vi "test-timer-all.vi"(8 "error in (no error)":errorcluster) -> (0 "error out":errorcluster, 3 "ALL TESTS PASSED":bool)   [LabVIEW 2019]
uses:
  <vilib>/Utility/semaphor.llb/Obtain Semaphore Reference.vi
  <vilib>/Rock Robotics/WPI/ThirdParty/JAS_Junk/TrajLib/Trajectory_Library.lvlib
panel:
  out "error out 2":errorcluster
  out "T5 - 2   0.500":dbl
  out "T5 Passed":bool
  out "T5 - 1":dbl
  out "T5 - 0":dbl
  out "T4 - 6 FALSE":bool
  out "T4 - 4 TRUE":bool
  out "T4 - 5 TRUE":bool
  out "T4 - 2 TRUE":bool
  out "T4 - 3 FALSE":bool
  out "T4 - 1 FALSE":bool
  out "T4 - 0 FALSE":bool
  out "T4 Passed":bool
  out "T3 Passed":bool
  out "T3-3 -- 0.0":dbl
  out "T3-2 -- 0.5":dbl
  out "T3-1 -- 0.0":dbl
  out "T3-0 -- 0.5":dbl
  out "Expired 2":bool
  out "Expired":bool
  out "T2 After Start":dbl
  out "Passed 2":bool
  out "T1 After Stop":dbl
  out "T1 After Start":dbl
  out "Passed 0A":bool
  out "Passed 0":bool
  out "T0 - Diff = 5.0":dbl
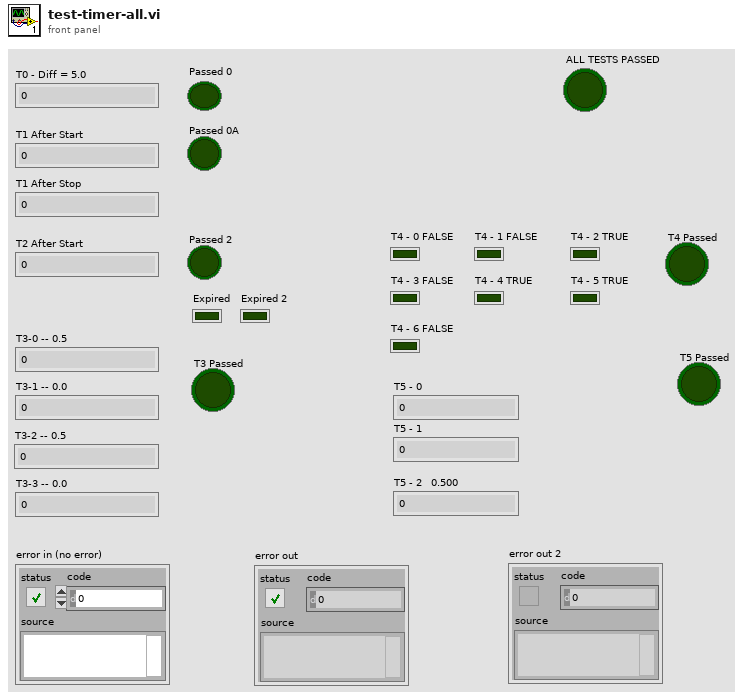
[diagram p1: front panel]
types:
  T1 = typedef "Trajectory_Library.lvlib/TIMER.ctl" = cluster{"StartTime":dbl, "Accumulated TIme":dbl, "Running":bool, "semaphore":T2}
  T2 = typedef "Semaphore RefNum" = refnum<k1>
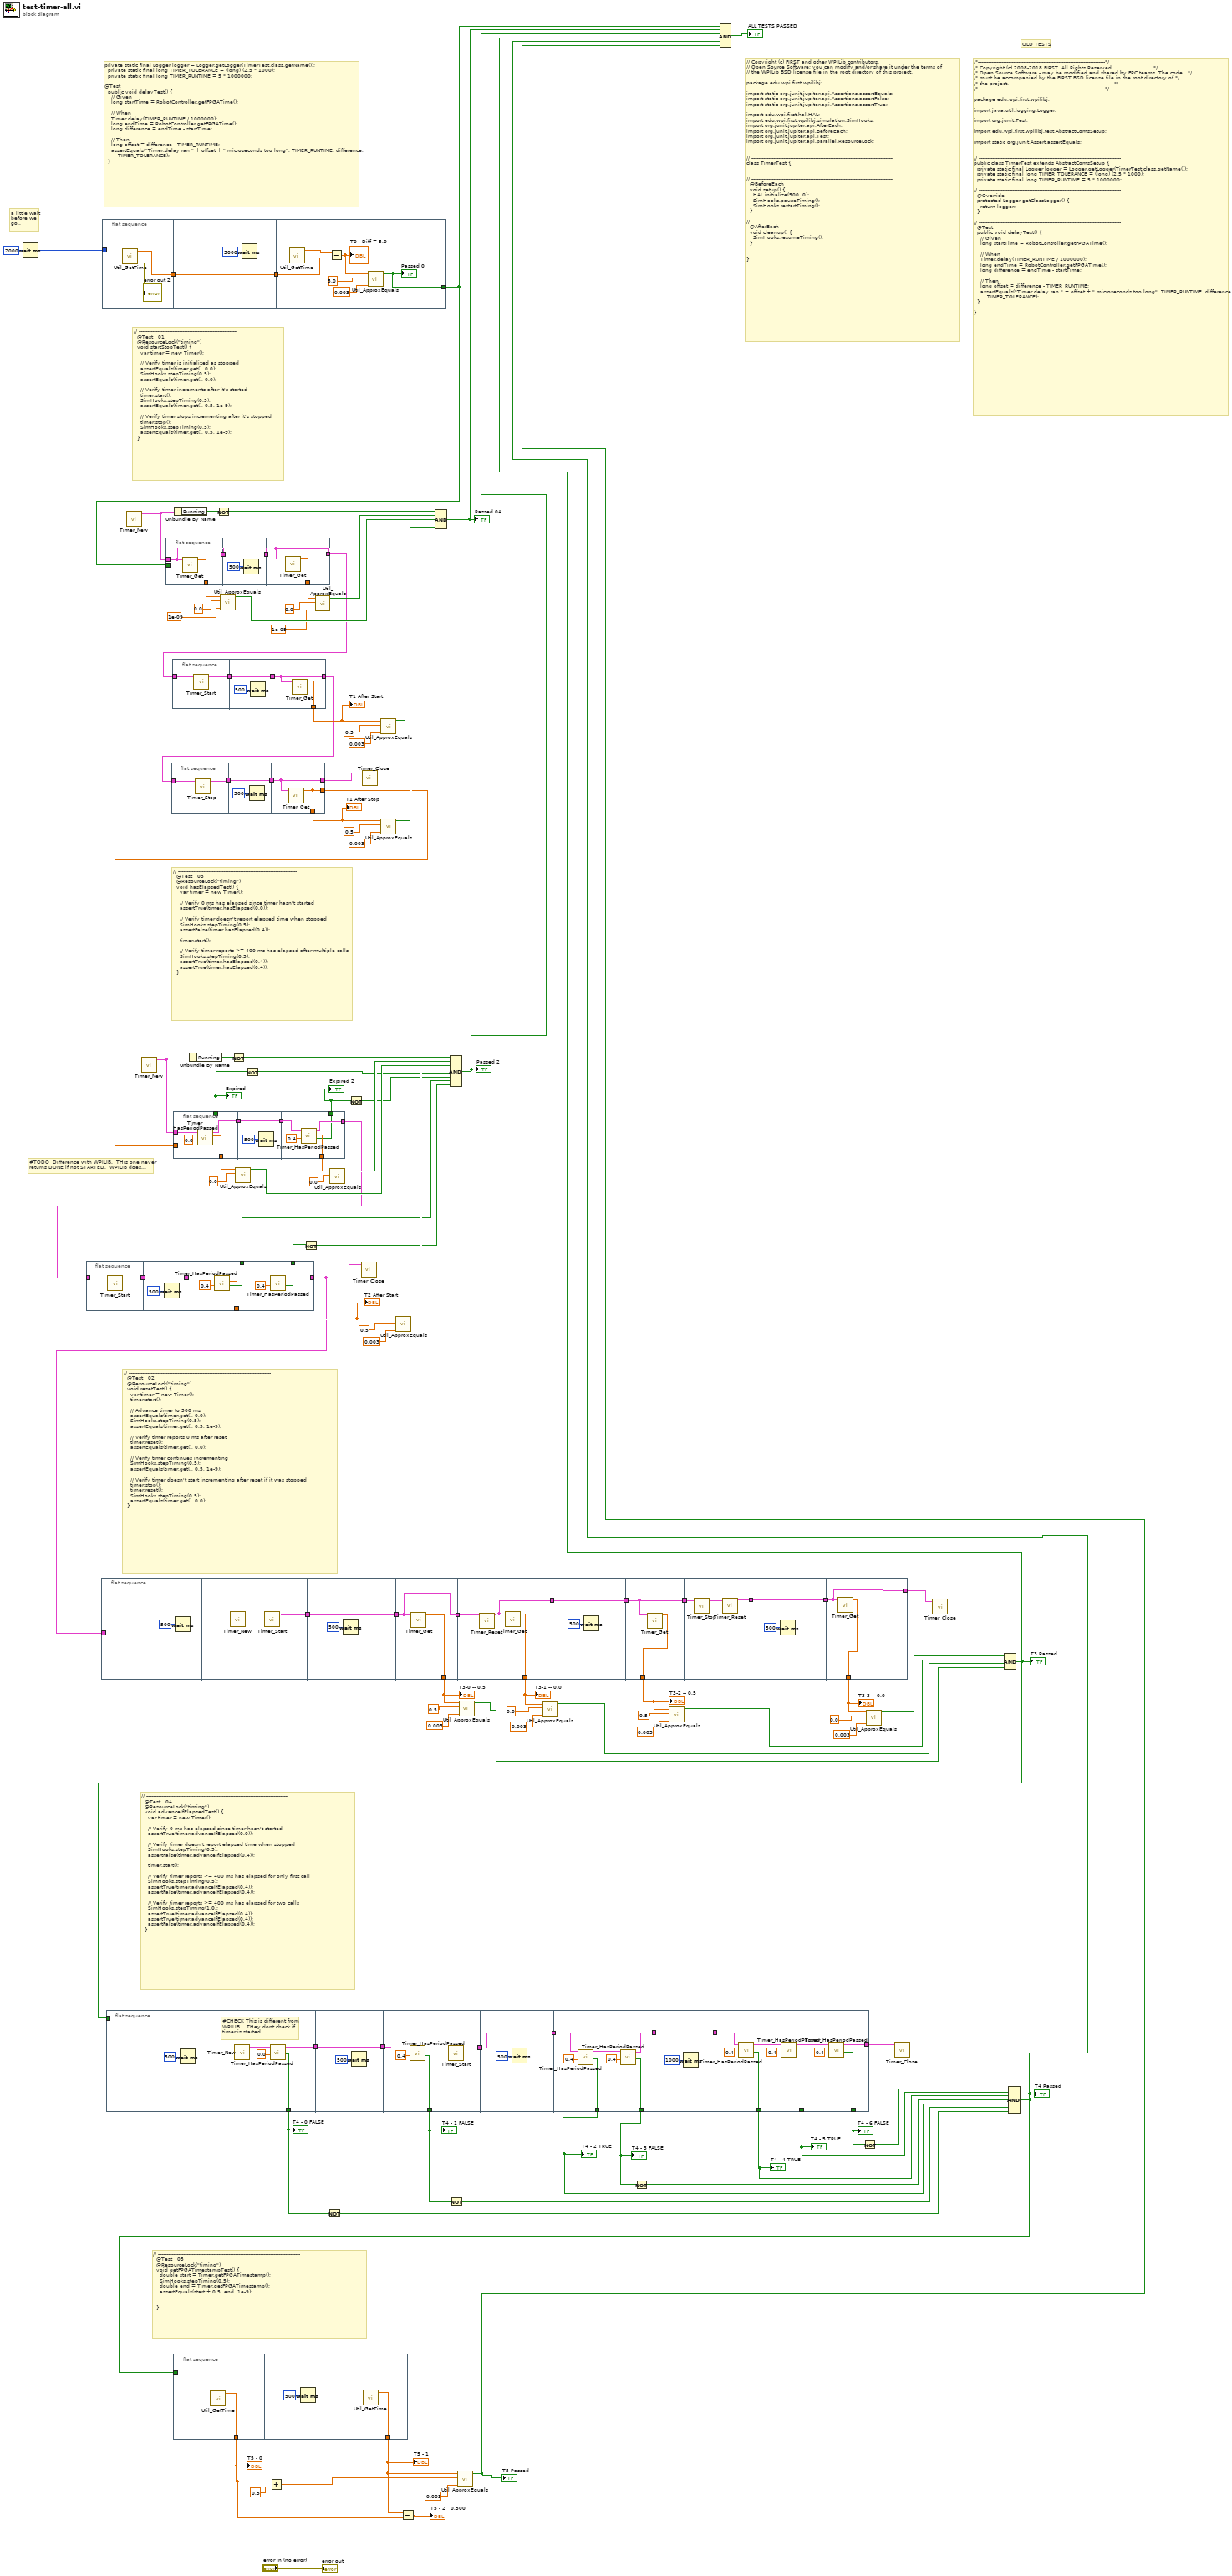
[diagram p0: block diagram]
diagram:
  # "// -------------------------------------------------------------------------------------\n  @Test   05\n  @ResourceLock(\"timing\")\n  void getFPGATimestampTest() {\n    double start = Timer.getFPGATimestamp();\n    SimHooks.stepTiming(0.5);\n    double end = Timer.getFPGATimestamp();\n    assertEquals(start + 0.5, end, 1e-9);\n\n\n  }"
  # "OLD TESTS"
  # "// -------------------------------------------------------------------------------------\n  @Test   04\n  @ResourceLock(\"timing\")\n  void advanceIfElapsedTest() {\n    var timer = new Timer();\n\n    // Verify 0 ms has elapsed since timer hasn't started\n    assertTrue(timer.advanceIfElapsed(0.0));\n\n    // Verify timer doesn't report elapsed time when stopped\n    SimHooks.stepTiming(0.5);\n    assertFalse(timer.advanceIfElapsed(0.4));\n\n    timer.start();\n\n    // Verify timer reports >= 400 ms has elapsed for only first call\n    SimHooks.stepTiming(0.5);\n    assertTrue(timer.advanceIfElapsed(0.4));\n    assertFalse(timer.advanceIfElapsed(0.4));\n\n    // Verify timer reports >= 400 ms has elapsed for two calls\n    SimHooks.stepTiming(1.0);\n    assertTrue(timer.advanceIfElapsed(0.4));\n    assertTrue(timer.advanceIfElapsed(0.4));\n    assertFalse(timer.advanceIfElapsed(0.4));\n  }"
  # "a little wait\nbefore we\ngo.."
  # "// -------------------------------------------------------------------------------------\n  @Test   02\n  @ResourceLock(\"timing\")\n  void resetTest() {\n    var timer = new Timer();\n    timer.start();\n\n    // Advance timer to 500 ms\n    assertEquals(timer.get(), 0.0);\n    SimHooks.stepTiming(0.5);\n    assertEquals(timer.get(), 0.5, 1e-9);\n\n    // Verify timer reports 0 ms after reset\n    timer.reset();\n    assertEquals(timer.get(), 0.0);\n\n    // Verify timer continues incrementing\n    SimHooks.stepTiming(0.5);\n    assertEquals(timer.get(), 0.5, 1e-9);\n\n    // Verify timer doesn't start incrementing after reset if it was stopped\n    timer.stop();\n    timer.reset();\n    SimHooks.stepTiming(0.5);\n    assertEquals(timer.get(), 0.0);\n  }"
  # "#TODO  Difference with WPILIB.  THis one never\nreturns DONE if not STARTED.  WPILIB does..."
  # "// -----------------------------------------------------------------------\n  @Test   03\n  @ResourceLock(\"timing\")\n  void hasElapsedTest() {\n    var timer = new Timer();\n\n    // Verify 0 ms has elapsed since timer hasn't started\n    assertTrue(timer.hasElapsed(0.0));\n\n    // Verify timer doesn't report elapsed time when stopped\n    SimHooks.stepTiming(0.5);\n    assertFalse(timer.hasElapsed(0.4));\n\n    timer.start();\n\n    // Verify timer reports >= 400 ms has elapsed after multiple calls\n    SimHooks.stepTiming(0.5);\n    assertTrue(timer.hasElapsed(0.4));\n    assertTrue(timer.hasElapsed(0.4));\n  }"
  # "// -----------------------------------------------------------\n  @Test   01\n  @ResourceLock(\"timing\")\n  void startStopTest() {\n    var timer = new Timer();\n\n    // Verify timer is initialized as stopped\n    assertEquals(timer.get(), 0.0);\n    SimHooks.stepTiming(0.5);\n    assertEquals(timer.get(), 0.0);\n\n    // Verify timer increments after it's started\n    timer.start();\n    SimHooks.stepTiming(0.5);\n    assertEquals(timer.get(), 0.5, 1e-9);\n\n    // Verify timer stops incrementing after it's stopped\n    timer.stop();\n    SimHooks.stepTiming(0.5);\n    assertEquals(timer.get(), 0.5, 1e-9);\n  }"
  # "/*----------------------------------------------------------------------------*/\n/* Copyright (c) 2008-2018 FIRST. All Rights Reserved.                        */\n/* Open Source Software - may be modified and shared by FRC teams. The code   */\n/* must be accompanied by the FIRST BSD license file in the root directory of */\n/* the project.                                                               */\n/*----------------------------------------------------------------------------*/\n\npackage edu.wpi.first.wpilibj;\n\nimport java.util.logging.Logger;\n\nimport org.junit.Test;\n\nimport edu.wpi.first.wpilibj.test.AbstractComsSetup;\n\nimport static org.junit.Assert.assertEquals;\n\n\n// -------------------------------------------------------------------------------------\npublic class TimerTest extends AbstractComsSetup {\n  private static final Logger logger = Logger.getLogger(TimerTest.class.getName());\n  private static final long TIMER_TOLERANCE = (long) (2.5 * 1000);\n  private static final long TIMER_RUNTIME = 5 * 1000000;\n\n// -------------------------------------------------------------------------------------\n  @Override\n  protected Logger getClassLogger() {\n    return logger;\n  }\n\n// -------------------------------------------------------------------------------------\n  @Test\n  public void delayTest() {\n    // Given\n    long startTime = RobotController.getFPGATime();\n\n    // When\n    Timer.delay(TIMER_RUNTIME / 1000000);\n    long endTime = RobotController.getFPGATime();\n    long difference = endTime - startTime;\n\n    // Then\n    long offset = difference - TIMER_RUNTIME;\n    assertEquals(\"Timer.delay ran \" + offset + \" microseconds too long\", TIMER_RUNTIME, difference,\n        TIMER_TOLERANCE);\n  }\n\n}"
  # "// Copyright (c) FIRST and other WPILib contributors.\n// Open Source Software; you can modify and/or share it under the terms of\n// the WPILib BSD license file in the root directory of this project.\n\npackage edu.wpi.first.wpilibj;\n\nimport static org.junit.jupiter.api.Assertions.assertEquals;\nimport static org.junit.jupiter.api.Assertions.assertFalse;\nimport static org.junit.jupiter.api.Assertions.assertTrue;\n\nimport edu.wpi.first.hal.HAL;\nimport edu.wpi.first.wpilibj.simulation.SimHooks;\nimport org.junit.jupiter.api.AfterEach;\nimport org.junit.jupiter.api.BeforeEach;\nimport org.junit.jupiter.api.Test;\nimport org.junit.jupiter.api.parallel.ResourceLock;\n\n\n// -------------------------------------------------------------------------------------\nclass TimerTest {\n\n\n// -------------------------------------------------------------------------------------\n  @BeforeEach\n  void setup() {\n    HAL.initialize(500, 0);\n    SimHooks.pauseTiming();\n    SimHooks.restartTiming();\n  }\n\n// -------------------------------------------------------------------------------------\n  @AfterEach\n  void cleanup() {\n    SimHooks.resumeTiming();\n  }\n\n\n}"
  # "private static final Logger logger = Logger.getLogger(TimerTest.class.getName());\n  private static final long TIMER_TOLERANCE = (long) (2.5 * 1000);\n  private static final long TIMER_RUNTIME = 5 * 1000000;\n\n@Test\n  public void delayTest() {\n    // Given\n    long startTime = RobotController.getFPGATime();\n\n    // When\n    Timer.delay(TIMER_RUNTIME / 1000000);\n    long endTime = RobotController.getFPGATime();\n    long difference = endTime - startTime;\n\n    // Then\n    long offset = difference - TIMER_RUNTIME;\n    assertEquals(\"Timer.delay ran \" + offset + \" microseconds too long\", TIMER_RUNTIME, difference,\n        TIMER_TOLERANCE);\n  }"
  n1 = Wait (ms)(milliseconds to wait=u32 2000) -> (millisecond timer value=w58:u32)
  n2 = flat-sequence {
    tunnel: w76 -> [w118]
    tunnel: [w117] -> w86
    tunnel: [w119] -> w85
    tunnel: w86 -> [w119]
    tunnel: [w121] -> w74
    tunnel: w85 -> [w128]
    tunnel: [w126] -> w57
    tunnel: [w123] -> w65
    tunnel: [w122] -> w64
    frame #0 {
      n3 = call <vilib>:"Timer_Start.vi"("in Timer"=w118) -> ("out Timer"=w117:T1)  [unwired: 10 in]
    }
    frame #1 {
      n4 = Wait (ms)(milliseconds to wait=u32 500) -> ()  [unwired: 1 out]
    }
    frame #2 {
      n5 = call <vilib>:"Timer_HasPeriodPassed.vi"("Period"=0.4, "in Timer"=w128) -> ("Expired"=w123:bool, "CurrentTImer"=w121:dbl, "out Timer"=w127:T1)  [unwired: 7 in]
      n6 = call <vilib>:"Timer_HasPeriodPassed.vi"("Period"=0.4, "in Timer"=w127) -> ("Expired"=w122:bool, "out Timer"=w126:T1)  [unwired: 7 in, 1 out]
    }
  }
  n7 = flat-sequence {
    tunnel: w57 -> [_]
    tunnel: [w130] -> w56
    tunnel: w56 -> [w132]
    tunnel: [w132] -> w55
    tunnel: w55 -> [w135]
    tunnel: [w135] -> w54
    tunnel: [w134] -> w51
    tunnel: w54 -> [w138]
    tunnel: [w137] -> w49
    tunnel: [w136] -> w46
    tunnel: [w139] -> w47
    tunnel: w46 -> [w139]
    tunnel: w47 -> [w141]
    tunnel: [w142] -> w43
    tunnel: [w141] -> w42
    tunnel: w42 -> [w144]
    tunnel: [w143] -> w40
    tunnel: [w146] -> w41
    tunnel: w40 -> [w146]
    tunnel: w41 -> [w148]
    tunnel: [w149] -> w37
    tunnel: [w148] -> w35
    frame #0 {
      n8 = Wait (ms)(milliseconds to wait=u32 500) -> ()  [unwired: 1 out]
    }
    frame #1 {
      n9 = call <vilib>:"Timer_New.vi"() -> ("TIMER"=w131:T1)  [unwired: 11 in]
      n10 = call <vilib>:"Timer_Start.vi"("in Timer"=w131) -> ("out Timer"=w130:T1)  [unwired: 10 in]
    }
    frame #2 {
      n11 = Wait (ms)(milliseconds to wait=u32 500) -> ()  [unwired: 1 out]
    }
    frame #3 {
      n12 = call <vilib>:"Timer_Get.vi"("TIMER"=w135) -> ("CurrentTImer"=w134:dbl)  [unwired: 10 in]
    }
    frame #4 {
      n13 = call <vilib>:"Timer_Reset.vi"("in TIMER"=w138) -> ("out TIMER"=w136:T1)  [unwired: 10 in]
      n14 = call <vilib>:"Timer_Get.vi"("TIMER"=w136) -> ("CurrentTImer"=w137:dbl)  [unwired: 10 in]
    }
    frame #5 {
      n15 = Wait (ms)(milliseconds to wait=u32 500) -> ()  [unwired: 1 out]
    }
    frame #6 {
      n16 = call <vilib>:"Timer_Get.vi"("TIMER"=w141) -> ("CurrentTImer"=w142:dbl)  [unwired: 10 in]
    }
    frame #7 {
      n17 = call <vilib>:"Timer_Stop.vi"("in Timer"=w144) -> ("out Timer"=w145:T1)  [unwired: 10 in]
      n18 = call <vilib>:"Timer_Reset.vi"("in TIMER"=w145) -> ("out TIMER"=w143:T1)  [unwired: 10 in]
    }
    frame #8 {
      n19 = Wait (ms)(milliseconds to wait=u32 500) -> ()  [unwired: 1 out]
    }
    frame #9 {
      n20 = call <vilib>:"Timer_Get.vi"("TIMER"=w148) -> ("CurrentTImer"=w149:dbl)  [unwired: 10 in]
    }
  }
  n21 = flat-sequence {
    tunnel: [w151] -> w116
    tunnel: w58 -> [_]
    tunnel: [w152] -> w115
    tunnel: w116 -> [w152]
    tunnel: w115 -> [w158]
    tunnel: [w154] -> w60
    frame #0 {
      n22 = call <vilib>:"Util_GetTime.vi"() -> ("error out"=→"error out 2":errorcluster, "FPGA_Time_Seconds"=w151:dbl)  [unwired: 10 in]
    }
    frame #1 {
      n23 = Wait (ms)(milliseconds to wait=u32 5000) -> ()  [unwired: 1 out]
    }
    frame #2 {
      n24 = call <vilib>:"Util_GetTime.vi"() -> ("FPGA_Time_Seconds"=w159:dbl)  [unwired: 10 in, 1 out]
      n25 = Subtract(x=w159, y=w158) -> (x-y=w157:dbl)
      "T0 - Diff = 5.0" <- w157
      n26 = call <vilib>:"Util_ApproxEquals.vi"("Tolerance"=0.003, "Value 2"=5.0, "Value 1"=w157) -> ("ApproxEquals"=w154:bool)  [unwired: 8 in]
      "Passed 0" <- w154
    }
  }
  n27 = flat-sequence {
    tunnel: w27 -> [_]
    tunnel: [w162] -> w30
    tunnel: [w161] -> w12
    tunnel: w30 -> [w165]
    tunnel: [w165] -> w29
    tunnel: w29 -> [w170]
    tunnel: [w169] -> w15
    tunnel: [w167] -> w26
    tunnel: [w172] -> w28
    tunnel: w26 -> [w172]
    tunnel: w28 -> [w178]
    tunnel: [w176] -> w16
    tunnel: [w175] -> w18
    tunnel: [w174] -> w25
    tunnel: w25 -> [w181]
    tunnel: [w181] -> w24
    tunnel: w24 -> [w189]
    tunnel: [w186] -> w22
    tunnel: [w185] -> w20
    tunnel: [w184] -> w19
    tunnel: [w183] -> w23
    frame #0 {
      n28 = Wait (ms)(milliseconds to wait=u32 500) -> ()  [unwired: 1 out]
    }
    frame #1 {
      # "#CHECK This is different from\nWPILIB .  THey dont check if\ntimer is started..."
      n29 = call <vilib>:"Timer_New.vi"() -> ("TIMER"=w164:T1)  [unwired: 11 in]
      n30 = call <vilib>:"Timer_HasPeriodPassed.vi"("Period"=0.0, "in Timer"=w164) -> ("Expired"=w161:bool, "out Timer"=w162:T1)  [unwired: 7 in, 1 out]
    }
    frame #2 {
      n31 = Wait (ms)(milliseconds to wait=u32 500) -> ()  [unwired: 1 out]
    }
    frame #3 {
      n32 = call <vilib>:"Timer_HasPeriodPassed.vi"("Period"=0.4, "in Timer"=w170) -> ("Expired"=w169:bool, "out Timer"=w168:T1)  [unwired: 7 in, 1 out]
      n33 = call <vilib>:"Timer_Start.vi"("in Timer"=w168) -> ("out Timer"=w167:T1)  [unwired: 10 in]
    }
    frame #4 {
      n34 = Wait (ms)(milliseconds to wait=u32 500) -> ()  [unwired: 1 out]
    }
    frame #5 {
      n35 = call <vilib>:"Timer_HasPeriodPassed.vi"("Period"=0.4, "in Timer"=w178) -> ("Expired"=w176:bool, "out Timer"=w177:T1)  [unwired: 7 in, 1 out]
      n36 = call <vilib>:"Timer_HasPeriodPassed.vi"("Period"=0.4, "in Timer"=w177) -> ("Expired"=w175:bool, "out Timer"=w174:T1)  [unwired: 7 in, 1 out]
    }
    frame #6 {
      n37 = Wait (ms)(milliseconds to wait=u32 1000) -> ()  [unwired: 1 out]
    }
    frame #7 {
      n38 = call <vilib>:"Timer_HasPeriodPassed.vi"("Period"=0.4, "in Timer"=w189) -> ("Expired"=w184:bool, "out Timer"=w190:T1)  [unwired: 7 in, 1 out]
      n39 = call <vilib>:"Timer_HasPeriodPassed.vi"("Period"=0.4, "in Timer"=w190) -> ("Expired"=w185:bool, "out Timer"=w187:T1)  [unwired: 7 in, 1 out]
      n40 = call <vilib>:"Timer_HasPeriodPassed.vi"("Period"=0.4, "in Timer"=w187) -> ("Expired"=w186:bool, "out Timer"=w183:T1)  [unwired: 7 in, 1 out]
    }
  }
  n41 = call <vilib>:"Timer_New.vi"() -> ("TIMER"=w112:T1)  [unwired: 11 in]
  n42 = call <vilib>:"Timer_New.vi"() -> ("TIMER"=w82:T1)  [unwired: 11 in]
  n43 = flat-sequence {
    tunnel: w112 -> [w193]
    tunnel: [w194] -> w110
    tunnel: [w193] -> w104
    tunnel: w60 -> [_]
    tunnel: [w195] -> w105
    tunnel: w104 -> [w195]
    tunnel: [w198] -> w111
    tunnel: w105 -> [w197]
    tunnel: [w197] -> w103
    frame #0 {
      n44 = call <vilib>:"Timer_Get.vi"("TIMER"=w193) -> ("CurrentTImer"=w194:dbl)  [unwired: 10 in]
    }
    frame #1 {
      n45 = Wait (ms)(milliseconds to wait=u32 500) -> ()  [unwired: 1 out]
    }
    frame #2 {
      n46 = call <vilib>:"Timer_Get.vi"("TIMER"=w197) -> ("CurrentTImer"=w198:dbl)  [unwired: 10 in]
    }
  }
  n47 = flat-sequence {
    tunnel: [w199] -> w96
    tunnel: w94 -> [w200]
    tunnel: [w201] -> w95
    tunnel: w96 -> [w201]
    tunnel: [w203] -> w90
    tunnel: w95 -> [w204]
    tunnel: [w204] -> w89
    tunnel: [w203] -> w71
    frame #0 {
      n48 = call <vilib>:"Timer_Stop.vi"("in Timer"=w200) -> ("out Timer"=w199:T1)  [unwired: 10 in]
    }
    frame #1 {
      n49 = Wait (ms)(milliseconds to wait=u32 500) -> ()  [unwired: 1 out]
    }
    frame #2 {
      n50 = call <vilib>:"Timer_Get.vi"("TIMER"=w204) -> ("CurrentTImer"=w203:dbl)  [unwired: 10 in]
    }
  }
  n51 = flat-sequence {
    tunnel: w103 -> [w206]
    tunnel: [w205] -> w101
    tunnel: [w207] -> w102
    tunnel: w101 -> [w207]
    tunnel: [w210] -> w99
    tunnel: w102 -> [w209]
    tunnel: [w209] -> w94
    frame #0 {
      n52 = call <vilib>:"Timer_Start.vi"("in Timer"=w206) -> ("out Timer"=w205:T1)  [unwired: 10 in]
    }
    frame #1 {
      n53 = Wait (ms)(milliseconds to wait=u32 500) -> ()  [unwired: 1 out]
    }
    frame #2 {
      n54 = call <vilib>:"Timer_Get.vi"("TIMER"=w209) -> ("CurrentTImer"=w210:dbl)  [unwired: 10 in]
    }
  }
  n55 = flat-sequence {
    tunnel: w82 -> [w214]
    tunnel: [w215] -> w81
    tunnel: [w212] -> w88
    tunnel: w71 -> [_]
    tunnel: [w211] -> w67
    tunnel: [w216] -> w87
    tunnel: w88 -> [w216]
    tunnel: w87 -> [w222]
    tunnel: [w221] -> w76
    tunnel: [w219] -> w70
    tunnel: [w218] -> w69
    frame #0 {
      n56 = call <vilib>:"Timer_HasPeriodPassed.vi"("Period"=0.0, "in Timer"=w214) -> ("Expired"=w211:bool, "CurrentTImer"=w215:dbl, "out Timer"=w212:T1)  [unwired: 7 in]
    }
    frame #1 {
      n57 = Wait (ms)(milliseconds to wait=u32 500) -> ()  [unwired: 1 out]
    }
    frame #2 {
      n58 = call <vilib>:"Timer_HasPeriodPassed.vi"("Period"=0.4, "in Timer"=w222) -> ("Expired"=w218:bool, "CurrentTImer"=w219:dbl, "out Timer"=w221:T1)  [unwired: 7 in]
    }
  }
  n59 = flat-sequence {
    tunnel: [w223] -> w4
    tunnel: w10 -> [_]
    tunnel: [w225] -> w7
    frame #0 {
      n60 = call <vilib>:"Util_GetTime.vi"() -> ("FPGA_Time_Seconds"=w223:dbl)  [unwired: 10 in, 1 out]
    }
    frame #1 {
      n61 = Wait (ms)(milliseconds to wait=u32 500) -> ()  [unwired: 1 out]
    }
    frame #2 {
      n62 = call <vilib>:"Util_GetTime.vi"() -> ("FPGA_Time_Seconds"=w225:dbl)  [unwired: 10 in, 1 out]
    }
  }
  n63 = Unbundle By Name(w112) -> ("Running"=w114:bool)
  n64 = Unbundle By Name(w82) -> ("Running"=w84:bool)
  n65 = Not(x=w114) -> (.not. x?=w113:bool)
  n66 = call <vilib>:"Util_ApproxEquals.vi"("Tolerance"=1e-09, "Value 2"=0.0, "Value 1"=w110) -> ("ApproxEquals"=w106:bool)  [unwired: 8 in]
  n67 = Not(x=w84) -> (.not. x?=w83:bool)
  n68 = call <vilib>:"Util_ApproxEquals.vi"("Value 2"=0.0, "Value 1"=w81) -> ("ApproxEquals"=w77:bool)  [unwired: 9 in]
  n69 = Not(x=w67) -> (.not. x?=w68:bool)
  n70 = Add(x=w4, y=0.5) -> (x+y=w6:dbl)
  n71 = Not(x=w64) -> (.not. x?=w63:bool)
  n72 = call <vilib>:"Util_ApproxEquals.vi"("Tolerance"=1e-09, "Value 2"=0.0, "Value 1"=w111) -> ("ApproxEquals"=w107:bool)  [unwired: 8 in]
  n73 = Not(x=w12) -> (.not. x?=w13:bool)
  n74 = call <vilib>:"Util_ApproxEquals.vi"("Value 2"=0.0, "Value 1"=w70) -> ("ApproxEquals"=w78:bool)  [unwired: 9 in]
  n75 = Not(x=w69) -> (.not. x?=w66:bool)
  n76 = call <vilib>:"Timer_Close.vi"("TIMER"=w57) -> ()  [unwired: 11 in]
  n77 = call <vilib>:"Timer_Close.vi"("TIMER"=w89) -> ()  [unwired: 11 in]
  n78 = call <vilib>:"Util_ApproxEquals.vi"("Tolerance"=0.003, "Value 2"=0.5, "Value 1"=w99) -> ("ApproxEquals"=w98:bool)  [unwired: 8 in]
  n79 = call <vilib>:"Util_ApproxEquals.vi"("Tolerance"=0.003, "Value 2"=0.5, "Value 1"=w90) -> ("ApproxEquals"=w91:bool)  [unwired: 8 in]
  n80 = call <vilib>:"Util_ApproxEquals.vi"("Tolerance"=0.003, "Value 2"=0.5, "Value 1"=w74) -> ("ApproxEquals"=w73:bool)  [unwired: 8 in]
  n81 = Subtract(x=w7, y=w4) -> (x-y=→"T5 - 2   0.500":dbl)
  n82 = Compound Arithmetic op=AND(w113, w107, w106, w98, w91) -> (w61:bool)
  "Passed 0A" <- w61
  n83 = Not(x=w15) -> (.not. x?=w14:bool)
  n84 = Compound Arithmetic op=AND(w83, w78, w77, w73, w68, w66, w65, w63) -> (w31:bool)
  "Passed 2" <- w31
  n85 = call <vilib>:"Util_ApproxEquals.vi"("Tolerance"=0.003, "Value 2"=w6, "Value 1"=w7) -> ("ApproxEquals"=w8:bool)  [unwired: 8 in]
  "T5 Passed" <- w8
  n86 = call <vilib>:"Util_ApproxEquals.vi"("Tolerance"=0.003, "Value 2"=0.5, "Value 1"=w51) -> ("ApproxEquals"=w32:bool)  [unwired: 8 in]
  n87 = call <vilib>:"Util_ApproxEquals.vi"("Tolerance"=0.003, "Value 2"=0.0, "Value 1"=w49) -> ("ApproxEquals"=w33:bool)  [unwired: 8 in]
  n88 = Not(x=w18) -> (.not. x?=w17:bool)
  n89 = call <vilib>:"Util_ApproxEquals.vi"("Tolerance"=0.003, "Value 2"=0.5, "Value 1"=w43) -> ("ApproxEquals"=w34:bool)  [unwired: 8 in]
  n90 = Not(x=w22) -> (.not. x?=w21:bool)
  n91 = call <vilib>:"Util_ApproxEquals.vi"("Tolerance"=0.003, "Value 2"=0.0, "Value 1"=w37) -> ("ApproxEquals"=w36:bool)  [unwired: 8 in]
  n92 = call <vilib>:"Timer_Close.vi"("TIMER"=w23) -> ()  [unwired: 11 in]
  n93 = call <vilib>:"Timer_Close.vi"("TIMER"=w35) -> ()  [unwired: 11 in]
  n94 = Compound Arithmetic op=AND(w36, w34, w33, w32) -> (w27:bool)
  "T3 Passed" <- w27
  n95 = Compound Arithmetic op=AND(w21, w20, w19, w17, w16, w14, w13) -> (w10:bool)
  "T4 Passed" <- w10
  n96 = Compound Arithmetic op=AND(w60, w61, w31, w27, w10, w8) -> (→"ALL TESTS PASSED":bool)
  "T1 After Start" <- w99
  "T1 After Stop" <- w90
  "T2 After Start" <- w74
  "Expired" <- w67
  "Expired 2" <- w69
  "T3-0 -- 0.5" <- w51
  "T3-1 -- 0.0" <- w49
  "T3-2 -- 0.5" <- w43
  "T3-3 -- 0.0" <- w37
  "T4 - 0 FALSE" <- w12
  "T4 - 1 FALSE" <- w15
  "T4 - 3 FALSE" <- w18
  "T4 - 2 TRUE" <- w16
  "T4 - 5 TRUE" <- w20
  "T4 - 4 TRUE" <- w19
  "T4 - 6 FALSE" <- w22
  "T5 - 0" <- w4
  "T5 - 1" <- w7
  "error out" <- "error in (no error)"
